vi "verify parameters in range.vi"(8 "error in (no error)":errorcluster, 11 "Simulated_CCD_Camera in":refnum<class "Sim_CCD.lvclass">) -> (0 "error out":errorcluster, 3 "Simulated_CCD_Camera out":refnum<class "Sim_CCD.lvclass">)   [LabVIEW 2018, in "Sim_CCD.lvclass"]
doc: "Verify if the parameters of the camera are in range\n\nThe operating parameters of the CCDs must be within a predefined range. This function verifies if the values provided for these parameters meet this specification. If not, ACS will not allow to start an exposure."
uses:
  Sim_CCD.lvclass
  Sim_CCD.lvclass/Sim_CCD.ctl
panel:
  out "new operation mode":T1
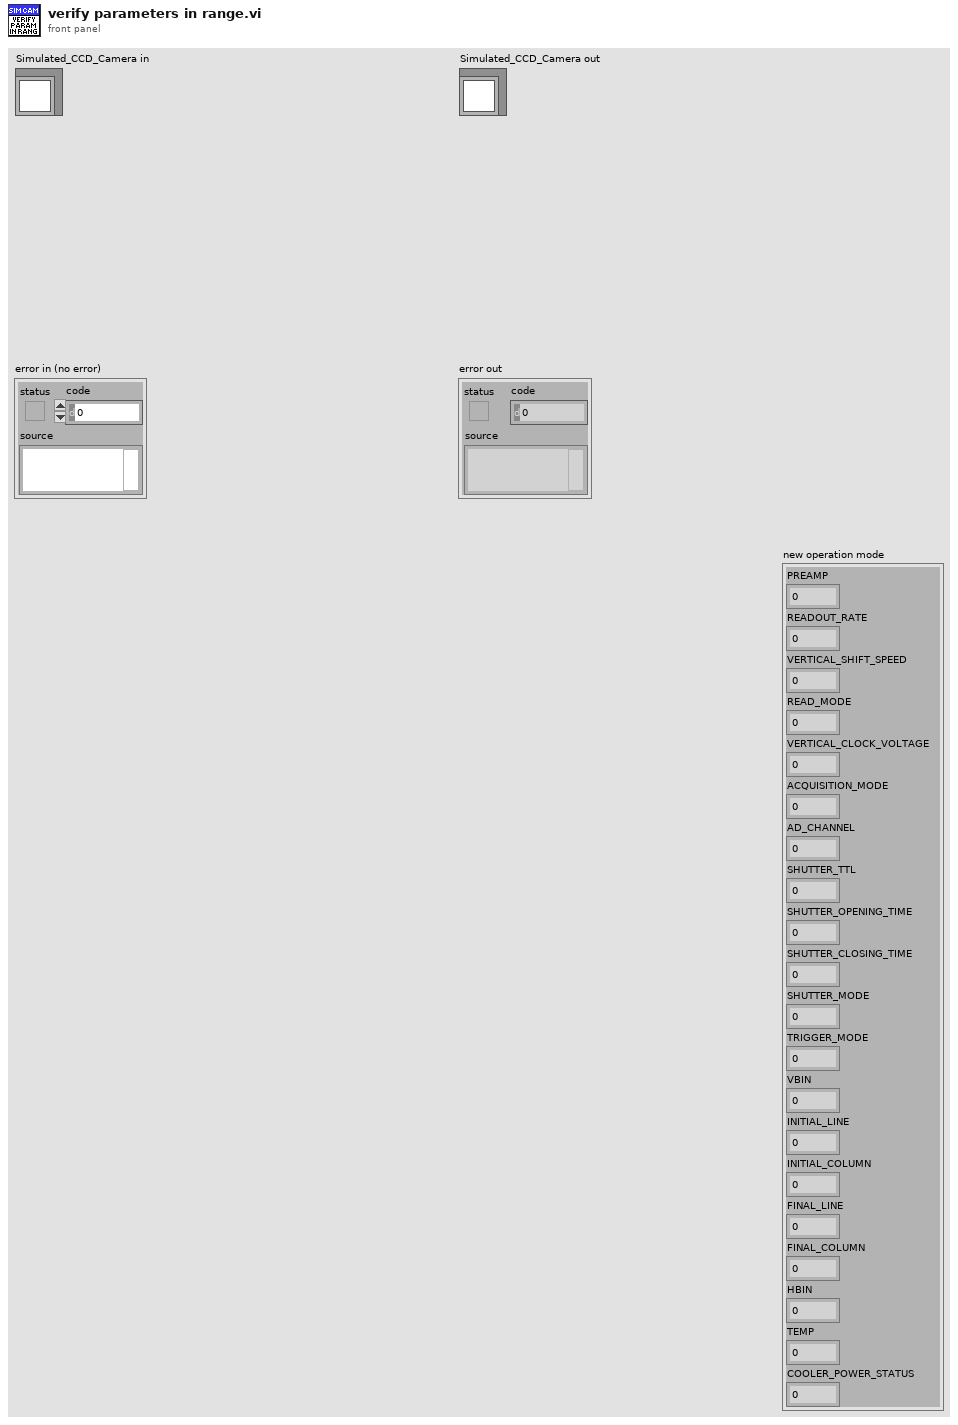
[diagram p1: front panel]
types:
  T1 = cluster{"PREAMP":u16, "READOUT_RATE":u16, "VERTICAL_SHIFT_SPEED":u16, "READ_MODE":u16, "VERTICAL_CLOCK_VOLTAGE":u16, "ACQUISITION_MODE":u16, "AD_CHANNEL":u16, "SHUTTER_TTL":u16, "SHUTTER_OPENING_TIME":u16, "SHUTTER_CLOSING_TIME":u16, "SHUTTER_MODE":u16, "TRIGGER_MODE":u16, "VBIN":u16, "INITIAL_LINE":u16, "INITIAL_COLUMN":u16, "FINAL_LINE":u16, "FINAL_COLUMN":u16, "HBIN":u16, "TEMP":i32, "COOLER_POWER_STATUS":u16}
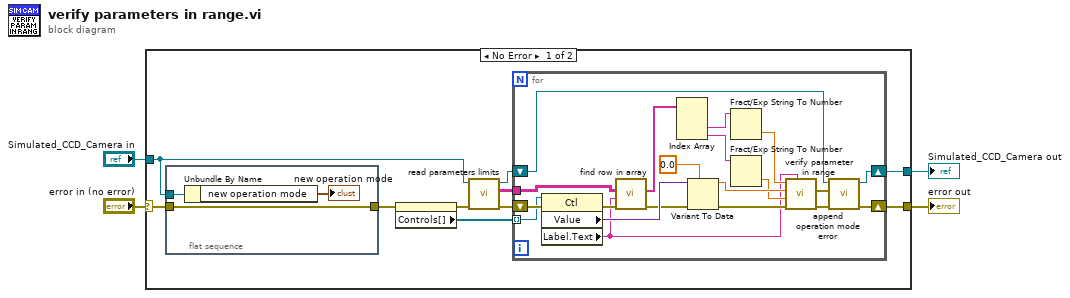
[diagram p0: block diagram]
diagram:
  n1 = case shown="No Error" "error in (no error)" {
    selector: "error in (no error)" -> [w8 w39]
    tunnel: [w14 w39] -> w3
    tunnel: [w13 w38] -> w2
    tunnel: "Simulated_CCD_Camera in" -> [w12 w38]
    frame No Error {
      n2 = flat-sequence {
        tunnel: w12 -> [w17]
        tunnel: w8 -> [w16]
        tunnel: [w16] -> w7
        frame #0 {
          n3 = Unbundle By Name(w17) -> ("new operation mode"=→"new operation mode":T1)
        }
      }
      n4 = property on="new operation mode" class="Clust (strict)"(error in=w7) -> (error out=w6:errorcluster, "Controls[]"=w5:refnum<vi>[])  [unwired: 1 in, 1 out]
      n5 = call "read parameters limits.vi"("error in (no error)"=w6, "Simulated_CCD_Camera in"=w12) -> ("error out"=w11:errorcluster, "limit values spreadsheet"=w10:string[][], "Simulated_CCD_Camera out"=w9:refnum<class "Sim_CCD.lvclass">)  [unwired: 7 in]
      n6 = for {
        shift-right: [w29] -> w14
        shift-left: w11 -> [w33]
        tunnel: w10 -> [w20]
        shift-right: [w25] -> w13
        shift-left: w9 -> [w18]
        tunnel: w5 -> [w32] mode=indexing
        n7 = property class="Ctl"(reference=w32, error in=w33) -> (error out=w22:errorcluster, "Value"=w37:variant, "Label.Text"=w19:string)  [unwired: 1 out]
        n8 = call "find row in array.vi"("error in (no error)"=w22, "parameter name"=w19, "limit values"=w20) -> ("error out"=w21:errorcluster, "row"=w23:string[])  [unwired: 7 in]
        n9 = Index Array(array=w23) -> (element #2=w35:string, element #3=w34:string)  [unwired: 3 in, 1 out]
        n10 = Variant To Data(error in=w21, type=0.0, Variant=w37) -> (data=w28:dbl, error out=w31:errorcluster)
        n11 = Fract/Exp String To Number(string=w35) -> (number=w27:dbl)  [unwired: 3 in, 1 out]
        n12 = Fract/Exp String To Number(string=w34) -> (number=w26:dbl)  [unwired: 3 in, 1 out]
        n13 = call "verify parameter in range.vi"("parameter name"=w19, "error in (no error)"=w31, "lower limit"=w26, "value"=w28, "upper limit"=w27) -> ("error out"=w30:errorcluster, "verific error"=w24:errorcluster)  [unwired: 5 in]
        n14 = call "append operation mode error.vi"("error in (no error)"=w30, "error"=w24, "Simulated_CCD_Camera in"=w18) -> ("error out"=w29:errorcluster, "Simulated_CCD_Camera out"=w25:refnum<class "Sim_CCD.lvclass">)  [unwired: 7 in]
      }
    }
    frame Error {
    }
  }
  "error out" <- w3
  "Simulated_CCD_Camera out" <- w2
